vi "Send Updated String.vi"(8 "error in (no error)":errorcluster, 10 "String Data":string, 11 "Nested Actor in":refnum<class "Nested Actor.lvclass">) -> (0 "error out":errorcluster, 3 "Nested Actor out":refnum<class "Nested Actor.lvclass">)   [LabVIEW 2018, in "Nested Actor.lvlib" / "Nested Actor.lvclass"]
uses:
  Nested Actor.lvclass
  C:/Program Files (x86)/National Instruments/LabVIEW 2018/vi.lib/ActorFramework/Actor/Actor.lvclass
  <vilib>/ActorFramework/Actor/Actor.lvclass/Actor.ctl
  Nested Actor.lvclass/Nested Actor.ctl
  Nested Actor Messages/New Data Msg/New Data Msg.lvclass/New Data Msg.ctl
  <vilib>/ActorFramework/Message Enqueuer/Message Enqueuer.lvclass/Message Enqueuer.ctl
  <vilib>/ActorFramework/Message Enqueuer/Enqueue.vi
  Nested Actor Messages/New Data Msg/New Data Msg.lvclass
  C:/Program Files (x86)/National Instruments/LabVIEW 2018/vi.lib/ActorFramework/Message/Message.lvclass
  <vilib>/ActorFramework/Message Priority Queue/Priority Enqueue.vi
  <vilib>/ActorFramework/Actor/Actor.lvclass
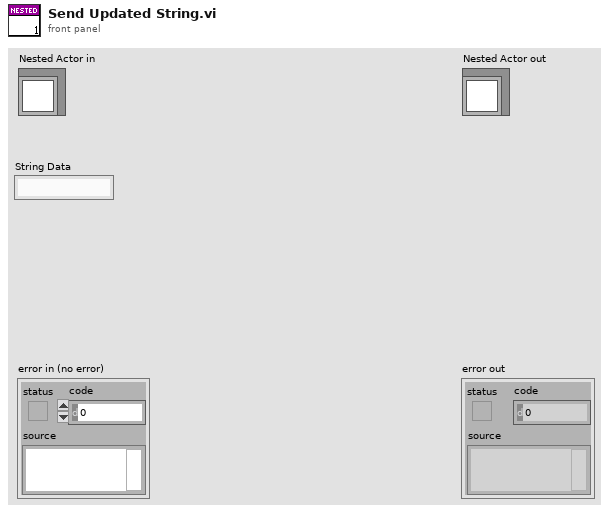
[diagram p1: front panel]
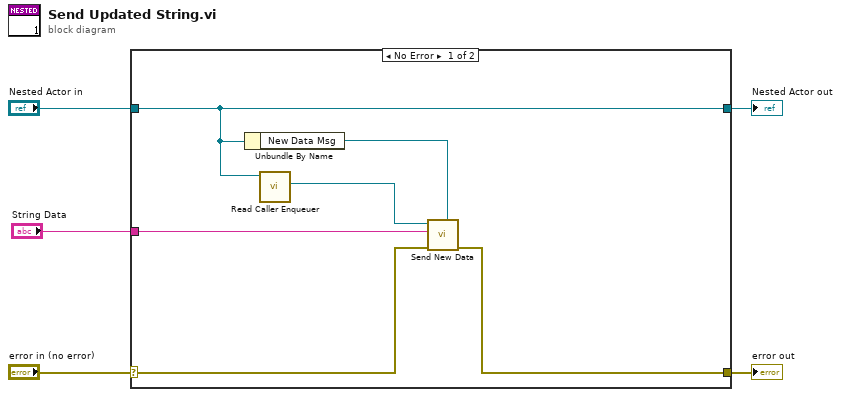
[diagram p0: block diagram]
diagram:
  n1 = case shown="No Error" "error in (no error)" {
    selector: "error in (no error)" -> [w7 w13]
    tunnel: [w6 w13] -> w4
    tunnel: [w9 w12] -> w2
    tunnel: "Nested Actor in" -> [w9 w12]
    tunnel: "String Data" -> [w10 _]
    frame No Error {
      n2 = Unbundle By Name(w9) -> ("New Data Msg"=w8:refnum<class "New Data Msg.lvclass">)
      n3 = call <vilib>:"Read Caller Enqueuer.vi"("Actor"=w9) -> ("Caller Enqueuer"=w11:refnum<class "Message Enqueuer.lvclass">)  [unwired: 10 in]
      n4 = call "Send New Data.vi"("Message Type"=w8, "error in (no error)"=w7, "String Data"=w10, "Message Enqueuer"=w11) -> ("error out"=w6:errorcluster)  [unwired: 6 in, 1 out]
    }
    frame Error {
    }
  }
  "error out" <- w4
  "Nested Actor out" <- w2
